vi "set_command_delay.vi"(8 "error in (no error)":errorcluster) -> (0 "error out":errorcluster)   [LabVIEW 2018]
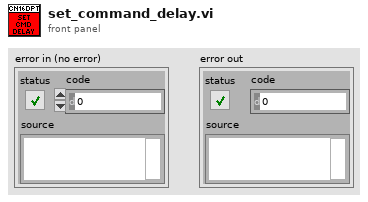
[diagram p1: front panel]
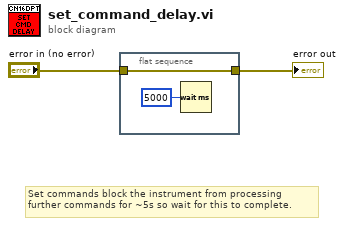
[diagram p0: block diagram]
diagram:
  # "Set commands block the instrument from processing\nfurther commands for ~5s so wait for this to complete."
  n1 = flat-sequence {
    tunnel: "error in (no error)" -> [w4]
    tunnel: [w4] -> w1
    frame #0 {
      n2 = Wait (ms)(milliseconds to wait=u32 5000) -> ()  [unwired: 1 out]
    }
  }
  "error out" <- w1
